vi "Actor Core.vi"(8 "error in":errorcluster, 11 "Splash Screen in":refnum<class "Splash Screen.lvclass">) -> (0 "error out":errorcluster, 3 "Actor out":refnum<class "Actor.lvclass">)   [LabVIEW 2018, in "Splash Screen.lvlib" / "Splash Screen.lvclass"]
doc: "(<B>Filename</B>: Actor Framework.lvlib:Actor.lvclass:Actor Core.vi)\n\nReceives messages to the actor, reacts to them, and initiates any error handling that may shut the actor down.\n\nDescendant classes may override this VI to append parallel tasks for the actor to complete while it handles messages. Overrides use the Call Parent Method node."
uses:
  Splash Screen.lvclass
  <vilib>/ActorFramework/Actor/Actor.lvclass
  Splash Screen.lvclass/Splash Screen.ctl
  UI Window/UI Window.lvclass
panel:
  out "Version":string
  in  "Stop?":bool
  out "Status Message":string
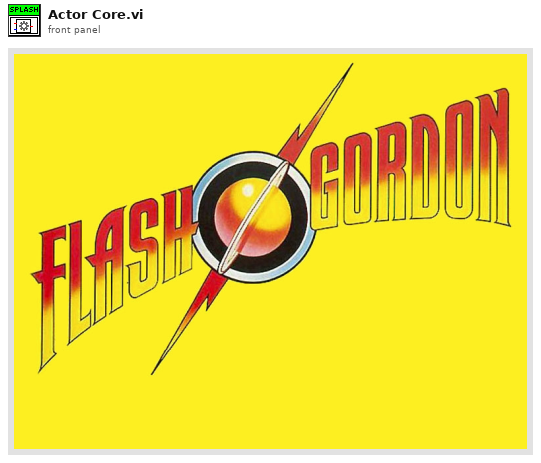
[diagram p1: front panel]
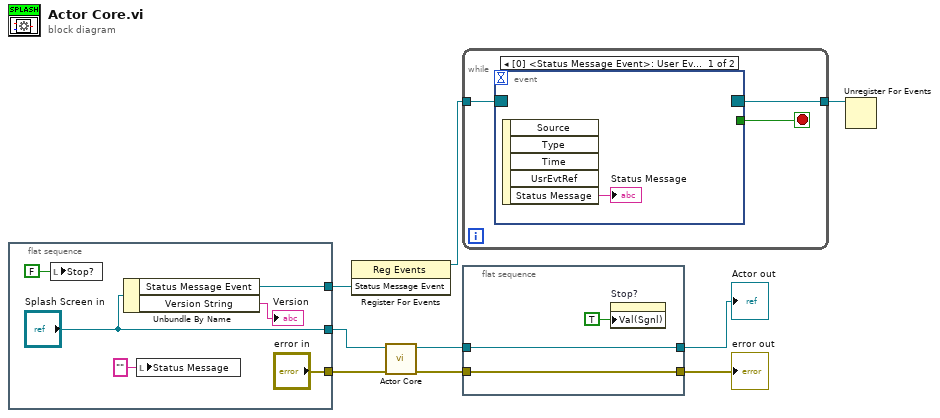
[diagram p0: block diagram]
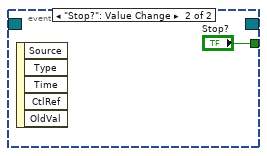
[diagram p2: hidden frame]
diagram:
  n1 = flat-sequence {
    tunnel: ["error in"] -> w9
    tunnel: [w13] -> w2
    tunnel: ["Splash Screen in"] -> w1
    frame #0 {
      n2 = local write "Stop?"(FALSE ("Stop?")) -> ()
      n3 = Unbundle By Name("Splash Screen in") -> ("Status Message Event"=w13:refnum<user-event>, "Version String"=→"Version":string)
      n4 = local write "Status Message"("" ("Status Message")) -> ()
    }
  }
  n5 = register-events(w2) -> (reference out=w8:refnum<event-registration>)  [unwired: 2 in, 1 out]
  n6 = call-parent "Actor Core.vi"("error in"=w9, "UI Window in"=w1) -> ("error out"=w6:errorcluster, "Actor out"=w7:refnum<class "Actor.lvclass">)  [unwired: 8 in]
  n7 = while {
    tunnel: w8 -> [w18]
    tunnel: [w16] -> w3
    stop <- w17 stop-if-true
    n8 = event shown="[0] <Status Message Event>: User Event" {
      selector: w18 -> [_ _]
      dyn-events: [_ _] -> w16
      timeout: _ -> [_ _]
      tunnel: [_ "Stop?"] -> w17
      event User Event {
        n9 = event-data() -> ("Status Message"=→"Status Message":string)  [unwired: 1 in, 4 out]
      }
      event "Stop?": Value Change {
        n10 = event-data() -> ()  [unwired: 1 in, 5 out]
      }
    }
  }
  n11 = flat-sequence {
    tunnel: w7 -> [w23]
    tunnel: w6 -> [w22]
    tunnel: [w23] -> w5
    tunnel: [w22] -> w4
    frame #0 {
      n12 = property on="Stop?" class="Bool (strict)"("Val(Sgnl)"=TRUE ("Stop?")) -> ()  [unwired: 2 in, 2 out]
    }
  }
  n13 = Unregister For Events(event registration refnum=w3) -> ()  [unwired: 1 in, 1 out]
  "Actor out" <- w5
  "error out" <- w4
